vi "Close.vi"(8 "error in (no error)":errorcluster, 10 "Msg in":T1, 11 "DG645 in":refnum<class "SMC100.lvclass">) -> (0 "error out":errorcluster, 1 "new command":string, 2 "Msg out":T1, 3 "DG645 out":refnum<class "SMC100.lvclass">)   [LabVIEW 2020, in "SMC100.lvclass"]
uses:
  SMC100.lvclass
  DriverMsg.ctl
  SMC100.lvclass/SMC100.ctl
  source/Device Drivers/BaseDriver/BaseDriver.lvclass
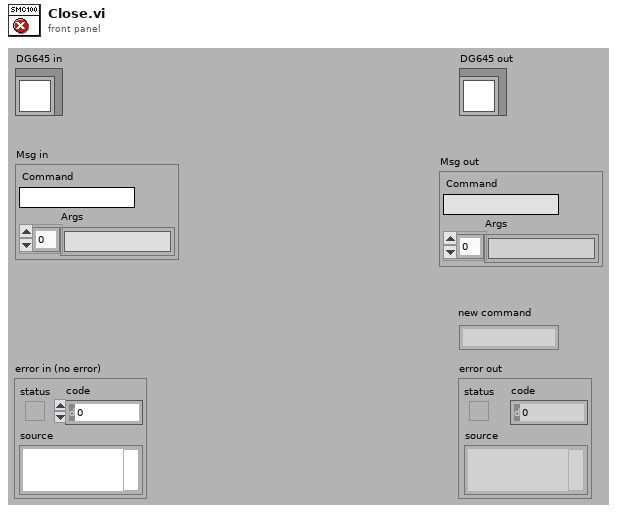
[diagram p1: front panel]
types:
  T1 = typedef "DriverMsg.ctl" = cluster{"Command":string, "Args":string[]}
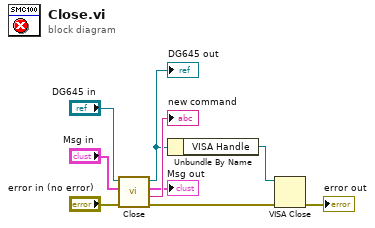
[diagram p0: block diagram]
diagram:
  n1 = call-parent "Close.vi"("error in (no error)"="error in (no error)", "Msg in"="Msg in", "BaseDriver in"="DG645 in") -> ("error out"=w2:errorcluster, "new command"=→"new command":string, "Msg out"=→"Msg out":T1, "BaseDriver out"=w4:refnum<class "SMC100.lvclass">)  [unwired: 5 in]
  "DG645 out" <- w4
  n2 = Unbundle By Name(w4) -> ("VISA Handle"=w3:refnum<visa-resource-name>)
  n3 = VISA Close(VISA resource name=w3, error in (no error)=w2) -> (error out=→"error out":errorcluster)
